vi "LVCAM Destroy Self.vi"(11 "Actor in":refnum<class "Actor.lvclass">) -> (0 "error out":errorcluster, 1 "Destroyed?":bool, 3 "Actor out":refnum<class "Actor.lvclass">)   [LabVIEW 2021, in "LVCAM.lvlib" / "Actor.lvclass"]
uses:
  Actor.lvclass
  C:/PPLs/LabVIEW-Composed-Actor-Model-LVCAM/LabVIEW-Composed-Actor-Model-LVCAM/LVCAM/LVCAM/LVCAM/LVCAM.lvclass
  Actor.lvclass/Actor.ctl
  State.ctl
  Msgs/LVCAM Destroy Self/LVCAM Destroy Self Msg/LVCAM Destroy Self Msg.lvclass
  C:/PPLs/LabVIEW-Composed-Actor-Model-LVCAM/LabVIEW-Composed-Actor-Model-LVCAM/LVCAM/LVCAM/Msg/Msg.lvclass
  Nest Msg Send.vi
  C:/PPLs/LabVIEW-Composed-Actor-Model-LVCAM/LabVIEW-Composed-Actor-Model-LVCAM/LVCAM/Msgs/LVCAM Create Nest/LVCAM Create Nest/LVCAM Create Nest.lvclass
  C:/PPLs/LabVIEW-Composed-Actor-Model-LVCAM/LabVIEW-Composed-Actor-Model-LVCAM/LVCAM/Msgs/LVCAM Destroy Self/LVCAM Destroy Self/LVCAM Destroy Self.lvclass
  C:/PPLs/LabVIEW-Composed-Actor-Model-LVCAM/LabVIEW-Composed-Actor-Model-LVCAM/LVCAM/Msgs/LVCAM Nest Destroyed/LVCAM Nest Destroyed/LVCAM Nest Destroyed.lvclass
  C:/PPLs/LabVIEW-Composed-Actor-Model-LVCAM/LabVIEW-Composed-Actor-Model-LVCAM/LVCAM/LVCAM/LVCAM Create/LVCAM Create.lvclass
  C:/PPLs/LabVIEW-Composed-Actor-Model-LVCAM/LabVIEW-Composed-Actor-Model-LVCAM/LVCAM/LVCAM/LVCAM Destroy/LVCAM Destroy.lvclass
  C:/PPLs/LabVIEW-Composed-Actor-Model-LVCAM/LabVIEW-Composed-Actor-Model-LVCAM/LVCAM/LVCAM/LVCAM Error/LVCAM Error.lvclass
  C:/PPLs/LabVIEW-Composed-Actor-Model-LVCAM/LabVIEW-Composed-Actor-Model-LVCAM/LVCAM/LVCAM/LVCAM Receive/LVCAM Receive.lvclass
  C:/PPLs/LabVIEW-Composed-Actor-Model-LVCAM/LabVIEW-Composed-Actor-Model-LVCAM/LVCAM/LVCAM/Actor/Actor.lvclass
  C:/PPLs/LabVIEW-Composed-Actor-Model-LVCAM/LabVIEW-Composed-Actor-Model-LVCAM/LVCAM/Msgs/LVCAM Destroy Self/LVCAM Destroy Self Msg/LVCAM Destroy Self Msg.lvclass
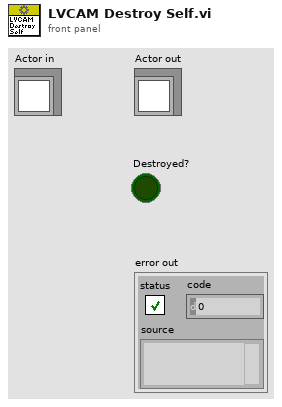
[diagram p1: front panel]
types:
  T1 = typedef "LVCAM.lvlib/Actor.lvclass/State.ctl" = enum16{"Msging", "Destroying"}
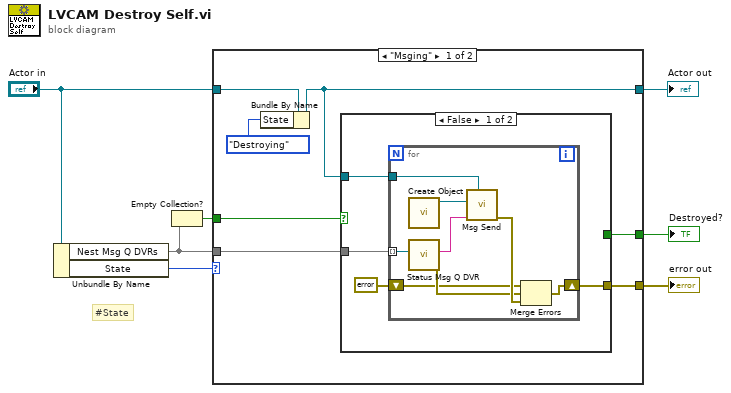
[diagram p0: block diagram]
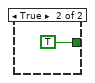
[diagram p2: hidden frame]
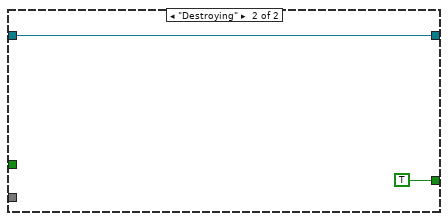
[diagram p3: hidden frame]
diagram:
  # "#State"
  n1 = Unbundle By Name("Actor in") -> ("Nest Msg Q DVRs"=w6:set{refnum<data-value>}, "State"=w1:T1)
  n2 = Empty Collection?(1:w6) -> (0:w7:bool)
  n3 = case shown="\"Msging\"" w1 {
    tunnel: w7 -> [w14 _]
    tunnel: w6 -> [w13 _]
    tunnel: [w12 TRUE ("Destroyed Self?")] -> w5
    tunnel: [w11 _] -> w4
    tunnel: [w8 w29] -> w3
    tunnel: "Actor in" -> [w9 w29]
    frame "Msging" {
      n4 = Bundle By Name(cluster=w9, "State"=State."Destroying") -> (w8:refnum<class "Actor.lvclass">)
      n5 = case shown="False" w14 {
        tunnel: w13 -> [w18 _]
        tunnel: [w17 _] -> w11
        tunnel: [_ TRUE ("Destroyed Self?")] -> w12
        tunnel: w8 -> [w15 _]
        frame False {
          n6 = for {
            tunnel: w18 -> [w22] mode=indexing
            shift-right: [w26] -> w17
            shift-left: errorcluster {"status"=FALSE, "code"=0, "source"=""} ("error out") -> [w19]
            tunnel: w15 -> [w23]
            n7 = call "Create Object.vi"() -> ("LVCAM Destroy Self Msg out"=w24:refnum<class "LVCAM Destroy Self Msg.lvclass">)  [unwired: 11 in]
            n8 = call "Status Msg Q DVR.vi"("Msg Q DVR"=w22) -> ("error out"=w20:errorcluster, "Msg Q DVR Alias"=w21:string)  [unwired: 9 in]
            n9 = call-poly "Msg Send.vi"("Actor"=w23, "Alias"=w21, "Msg"=w24) -> ("error out"=w25:errorcluster)  [unwired: 7 in, 1 out]
            n10 = Merge Errors(w19, w20, w25) -> (w26:errorcluster)
          }
        }
        frame True {
        }
      }
    }
    frame "Destroying" {
    }
  }
  "error out" <- w4
  "Actor out" <- w3
  "Destroyed?" <- w5
